vi "SwTmr Incorporate New Data.vi"(8 "error in (no error)":errorcluster, 10 "New Graph Data":waveform(dbl)[](array[waveform]), 11 "Data in":T1={"UI References"={"Stop Ref"=refnum, "Save Ref"=refnum, "Open Ref"=refnum, "Export Ref"=refnum, "Acquire Ref"=refnum, "Configure Ref"=refnum, "Graph Ref"=refnum, "Clear Ref"=refnum, "Analyze Ref"=refnum, "Status Ref"=refnum, "Snapshot Ref"=refnum}, "Graph Data"={"Data"=[], "Annotation List"=[], "Cursor List"=[], "Analysis Data"=[]}, "User Specified"={"Hardware Configuration"={"Physical Channel"="", "Maximum Input"=0.0, "Minimum Input"=0.0, "Sample Rate"=0.0, "Number of Samples"=0}, "Analysis Configuration"={"Statistics"=TRUE}, "New Data Behavior"=enum."Replace", "Time-Voltage transfer function file path (dialog if empty)"=path "", "Cell (V) Error Upper"=0.0, "Cell (V) Error Lower (type \"-\")"=0.0}}) -> (0 "error out":errorcluster, 3 "Data out":T1={"UI References"={"Stop Ref"=refnum, "Save Ref"=refnum, "Open Ref"=refnum, "Export Ref"=refnum, "Acquire Ref"=refnum, "Configure Ref"=refnum, "Graph Ref"=refnum, "Clear Ref"=refnum, "Analyze Ref"=refnum, "Status Ref"=refnum, "Snapshot Ref"=refnum}, "Graph Data"={"Data"=[], "Annotation List"=[], "Cursor List"=[], "Analysis Data"=[]}, "User Specified"={"Hardware Configuration"={"Physical Channel"="", "Maximum Input"=0.0, "Minimum Input"=0.0, "Sample Rate"=0.0, "Number of Samples"=0}, "Analysis Configuration"={"Statistics"=TRUE}, "New Data Behavior"=enum."Replace", "Time-Voltage transfer function file path (dialog if empty)"=path "", "Cell (V) Error Upper"=0.0, "Cell (V) Error Lower (type \"-\")"=0.0}})   [LabVIEW 2017]
doc: "Incorporates newly acquired or loaded data into the main state data. New data can replace, be appended to, or overlayed over (as an additional channel) existing data. If the user does not have a preference saved a dialog will be presented asking which method to use."
uses:
  controls/SwTmr Data.ctl
  controls/SwTmr UI References.ctl
  controls/SwTmr Graph Data.ctl
  <vilib>/Utility/miscctls.llb/LVAnnotationListTypeDef.ctl
  <vilib>/Utility/miscctls.llb/LVCursorListTypeDef.ctl
  controls/SwTmr User Specified Data.ctl
  controls/SwTmr HW Configuration.ctl
  controls/SwTmr Analysis Configuration.ctl
  controls/SwTmr New Data Behavior.ctl
  controls/SwTmr Transfer Func File Path.ctl
panel:
  # "(Scroll up to see large state data in/out clusters)"
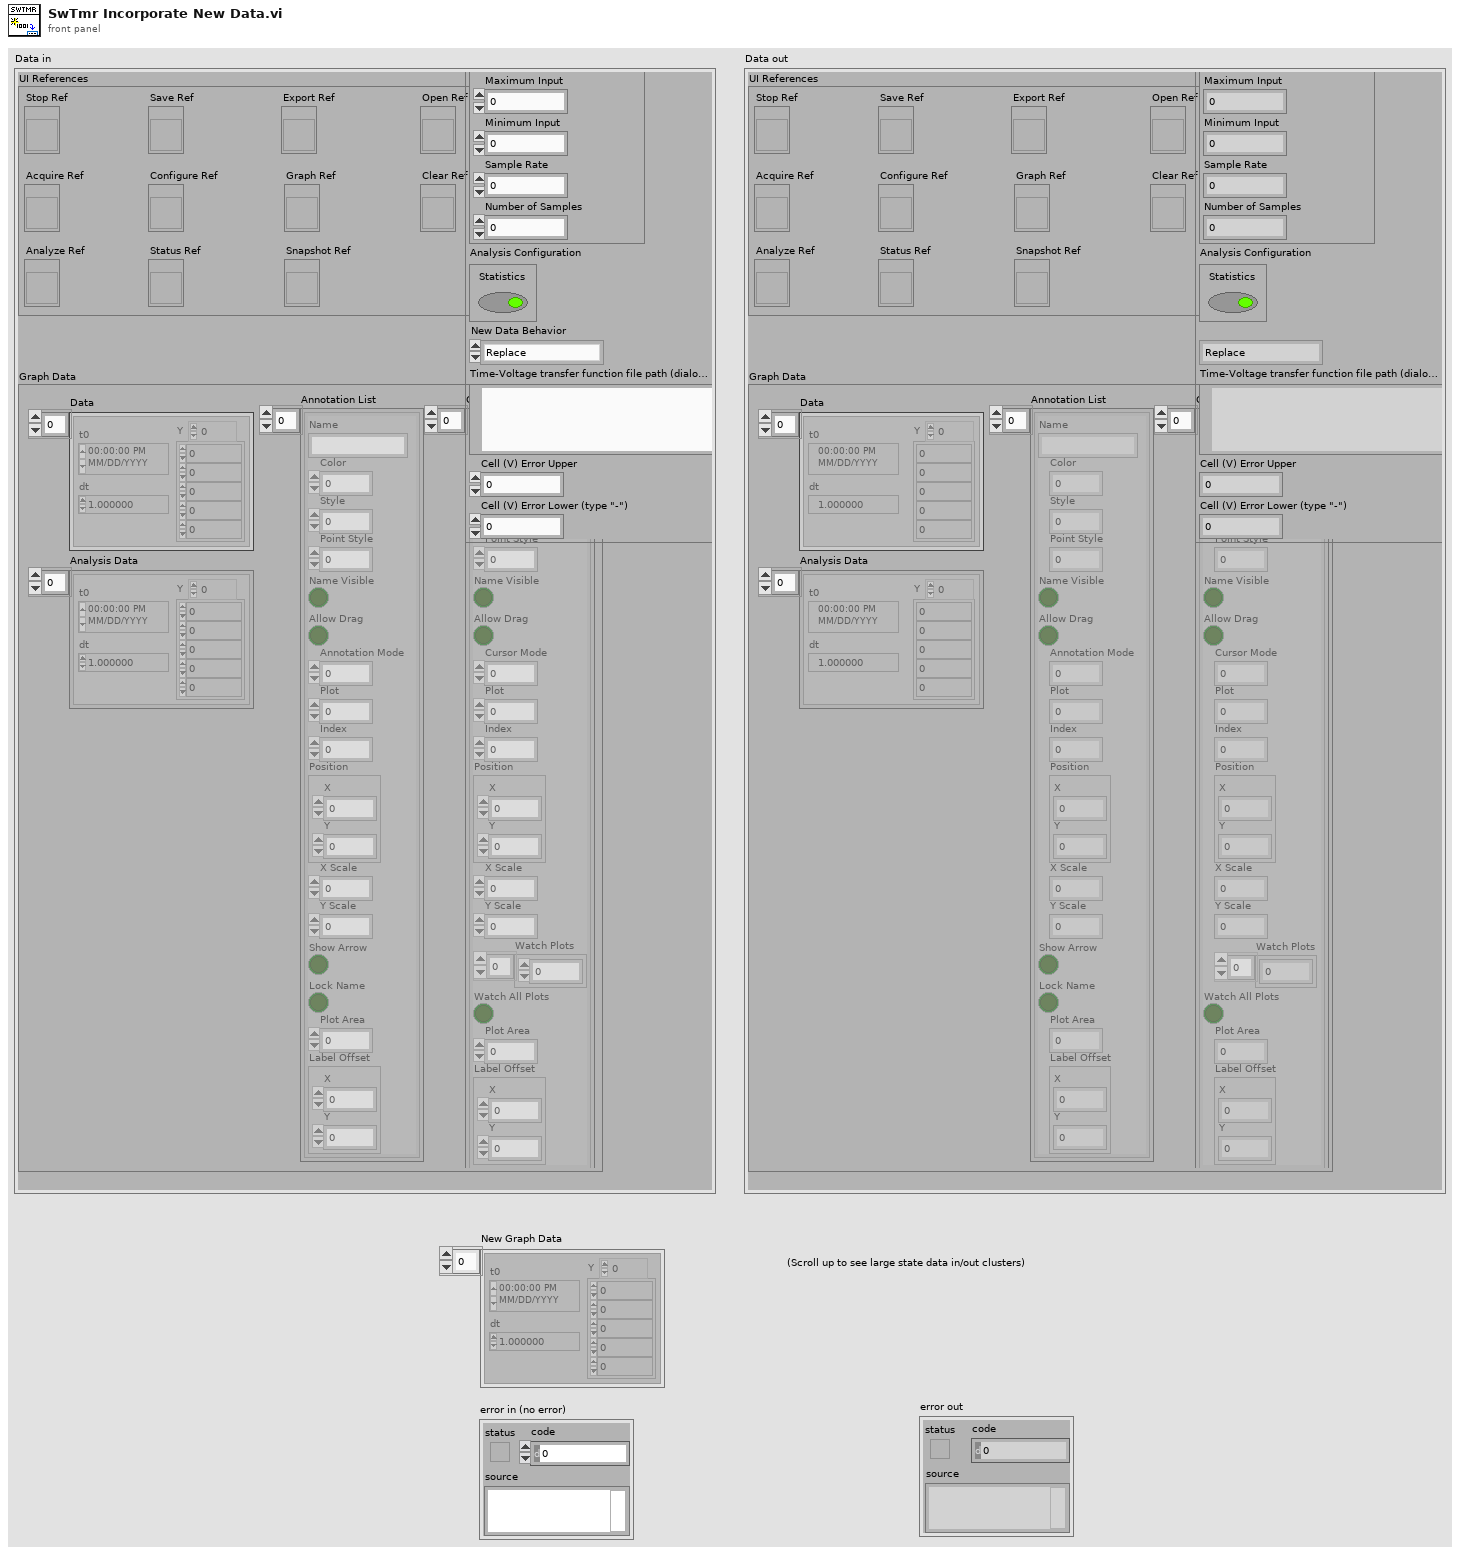
[diagram p1: front panel]
types:
  T1 = typedef "SwTmr Data.ctl" = cluster{"UI References":T2, "Graph Data":T3, "User Specified":T6}
  T2 = typedef "SwTmr UI References.ctl" = cluster{"Stop Ref":refnum<vi>, "Save Ref":refnum<vi>, "Open Ref":refnum<vi>, "Export Ref":refnum<vi>, "Acquire Ref":refnum<vi>, "Configure Ref":refnum<vi>, "Graph Ref":refnum<vi>, "Clear Ref":refnum<vi>, "Analyze Ref":refnum<vi>, "Status Ref":refnum<vi>, "Snapshot Ref":refnum<vi>}
  T3 = typedef "SwTmr Graph Data.ctl" = cluster{"Data":waveform(dbl)[], "Annotation List":T4, "Cursor List":T5, "Analysis Data":waveform(dbl)[]}
  T4 = typedef "LVAnnotationListTypeDef.ctl" = cluster{"Name":string, "Color":u32, "Style":u8, "Point Style":u8, "Name Visible":bool, "Allow Drag":bool, "Annotation Mode":u32, "Plot":i32, "Index":i32, "Position":cluster{"X":dbl, "Y":dbl}, "X Scale":u32, "Y Scale":u32, "Show Arrow":bool, "Lock Name":bool, "Plot Area":i32, "Label Offset":cluster{"X":dbl, "Y":dbl}}[]
  T5 = typedef "LVCursorListTypeDef.ctl" = cluster{"Name":string, "Color":u32, "Style":u8, "Point Style":u8, "Name Visible":bool, "Allow Drag":bool, "Cursor Mode":u32, "Plot":i32, "Index":i32, "Position":cluster{"X":dbl, "Y":dbl}, "X Scale":u32, "Y Scale":u32, "Watch Plots":i32[], "Watch All Plots":bool, "Plot Area":i32, "Label Offset":cluster{"X":dbl, "Y":dbl}}[]
  T6 = typedef "SwTmr User Specified Data.ctl" = cluster{"Hardware Configuration":T7, "Analysis Configuration":T8, "New Data Behavior":T9, "Time-Voltage transfer function file path (dialog if empty)":T10, "Cell (V) Error Upper":dbl, "Cell (V) Error Lower (type \"-\")":dbl}
  T7 = typedef "SwTmr HW Configuration.ctl" = cluster{"Physical Channel":tag, "Maximum Input":dbl, "Minimum Input":dbl, "Sample Rate":dbl, "Number of Samples":i32}
  T8 = typedef "SwTmr Analysis Configuration.ctl" = cluster{"Statistics":bool}
  T9 = typedef "SwTmr New Data Behavior.ctl" = enum16{"Replace", "Overlay", "Append"}
  T10 = typedef "SwTmr Transfer Func File Path.ctl" = path
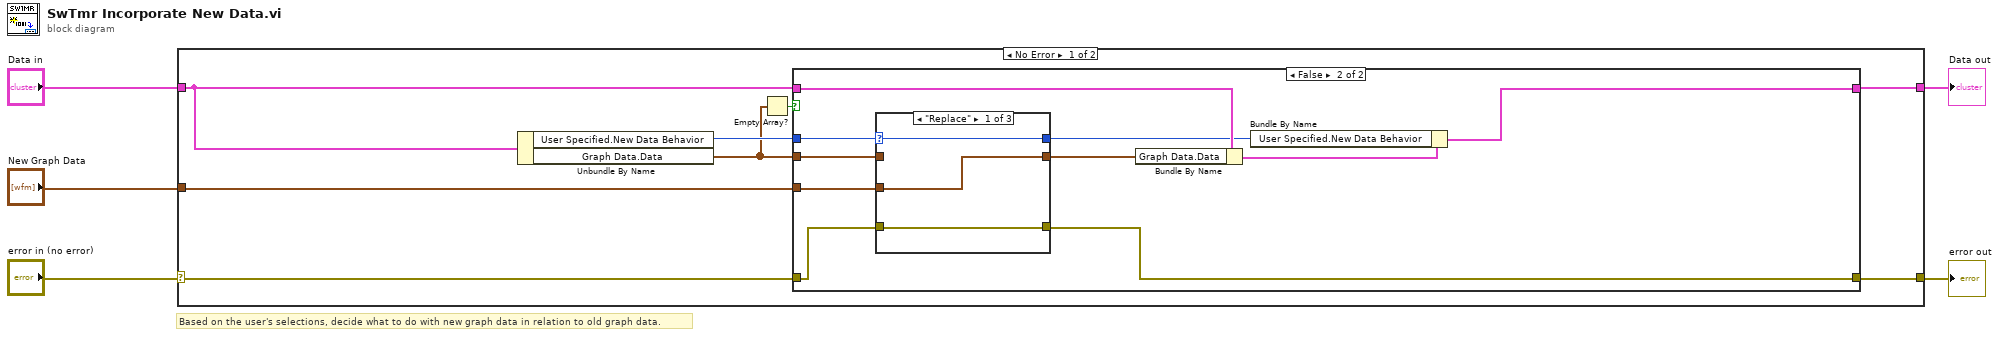
[diagram p0: block diagram]
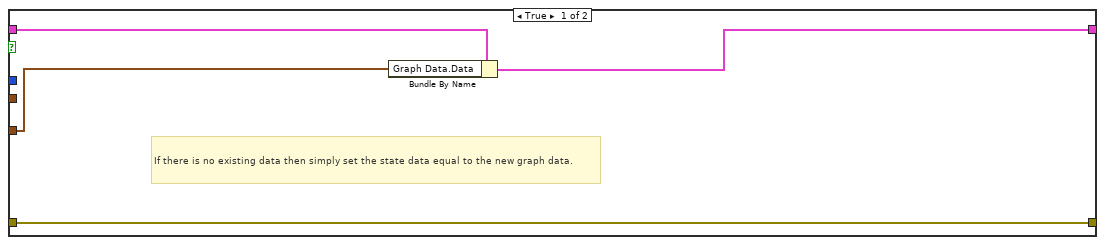
[diagram p2: hidden frame]
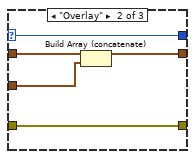
[diagram p3: hidden frame]
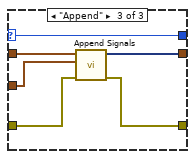
[diagram p4: hidden frame]
diagram:
  # "Based on the user's selections, decide what to do with new graph data in relation to old graph data."
  n1 = case shown="No Error" "error in (no error)" {
    selector: "error in (no error)" -> [w9 w43]
    tunnel: "Data in" -> [w13 w42]
    tunnel: "New Graph Data" -> [w11 _]
    tunnel: [w10 w42] -> w3
    tunnel: [w8 w43] -> w1
    frame No Error {
      n2 = Unbundle By Name(w13) -> ("User Specified.New Data Behavior"=w12:T9, "Graph Data.Data"=w7:waveform(dbl)[])
      n3 = Empty Array?(array=w7) -> (empty?=w6:bool)
      n4 = case shown="False" w6 {
        tunnel: w13 -> [w17 w27]
        tunnel: w12 -> [_ w26]
        tunnel: w11 -> [w16 w25]
        tunnel: w7 -> [_ w23]
        tunnel: [w15 w20] -> w10
        tunnel: w9 -> [w14 w19]
        tunnel: [w14 w18] -> w8
        frame True {
          # "If there is no existing data then simply set the state data equal to the new graph data."
          n5 = Bundle By Name(cluster=w17, "Graph Data.Data"=w16) -> (w15:T1)
        }
        frame False {
          n6 = case shown="\"Replace\"" w26 {
            selector: w26 -> [w29 w35 w38]
            tunnel: w25 -> [w30 w33 w40]
            tunnel: [w30 w32 w39] -> w24
            tunnel: [w29 w35 w38] -> w22
            tunnel: w23 -> [_ w34 w41]
            tunnel: w19 -> [w28 w31 w37]
            tunnel: [w28 w31 w36] -> w18
            frame "Replace" {
            }
            frame "Overlay" {
              n7 = Build Array (concatenate)(w34, w33) -> (w32:waveform(dbl)[])
            }
            frame "Append" {
              n8 = call "Append Signals"("error in (no error)"=w37, "Input Signal B"=w40, "Input Signal A"=w41) -> ("error out"=w36:errorcluster, "Appended Signals"=w39:dynamicdata)  [unwired: 7 in]
            }
          }
          n9 = Bundle By Name(cluster=w27, "Graph Data.Data"=w24) -> (w21:T1)
          n10 = Bundle By Name(cluster=w21, "User Specified.New Data Behavior"=w22) -> (w20:T1)
        }
      }
    }
    frame Error {
    }
  }
  "Data out" <- w3
  "error out" <- w1
